vi "Periodic Tasks.vi"(8 "error in":errorcluster) -> ()   [LabVIEW 2013]
doc: "This VI runs in parallel to other tasks. It can contain as many user-defined periodic loops as you need. These can carry out PID or other sorts of timed response."
uses:
  <vilib>/Rock Robotics/SystemInterfaces/DIO/FPGA_DIOChannel.ctl
  <vilib>/Rock Robotics/SystemInterfaces/DIO/FPGA_DIORelayChannel.ctl
  <vilib>/Rock Robotics/SystemInterfaces/Utilities/FPGA_UtilitiesLED Source.ctl
  <vilib>/Rock Robotics/SystemInterfaces/Utilities/FPGA_UtilitiesLED State.ctl
  871/Utils/Targetsss.ctl
  871/Utils/Target Type.ctl
  871/Utils/Scores.ctl
  <vilib>/Rock Robotics/WPI/Counter/WPI_CounterDigitalInputToDigitalSource.vi
  Robot Global Data.vi
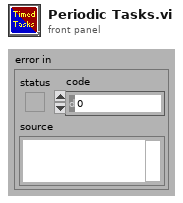
[diagram p1: front panel]
types:
  T1 = typedef "FPGA_DIORelayChannel.ctl" = enum8{"Relay 1", "Relay 2", "Relay 3", "Relay 4", "Relay 5", "Relay 6", "Relay 7", "Relay 8", "Invalid"}
  T2 = typedef "FPGA_DIOChannel.ctl" = enum8{"DIO 1", "DIO 2", "DIO 3", "DIO 4", "DIO 5", "DIO 6", "DIO 7", "DIO 8", "DIO 9", "DIO 10", "DIO 11", "DIO 12", "DIO 13", "DIO 14", "Invalid"}
  T3 = typedef "WPI_DigitalInputDevRef.ctl" = cluster{"DevStatus":errorcluster, "DIO Channel":T2, "Digital Module":T4}
  T4 = typedef "FPGA_TypedefDigitalModule.ctl" = enum16{"Digital Module 1", "Digital Module 2"}
  T5 = typedef "FPGA_CounterEncoderSourceConvertionLVSourceType.ctl" = cluster{"DevStatus":errorcluster, "AnalogTriggerMode?":bool, "DigitalMode":cluster{"Digital Module":T4, "DIO Channel":T6}, "AnalogTriggerMode":cluster{"AnalogTriggerIndex":T7, "OutputType":T8}}
  T6 = typedef "FPGA_DIODigitalSourceChannel.ctl" = enum8{"DIO 1", "DIO 2", "DIO 3", "DIO 4", "DIO 5", "DIO 6", "DIO 7", "DIO 8", "DIO 9", "DIO 10", "DIO 11", "DIO 12", "DIO 13", "DIO 14", "Disabled"}
  T7 = typedef "FPGA_AnalogTriggerIndex.ctl" = enum8{"Trig 0", "Trig 1", "Trig 2", "Trig 3", "Trig 4", "Trig 5", "Trig 6", "Trig 7", "Invalid"}
  T8 = typedef "FPGA_AnalogTriggerOutType.ctl" = enum16{"InWindow", "TriggerState", "Rising", "Falling"}
  T9 = typedef "WPI_InterruptRef.ctl" = cluster{"DevStatus":errorcluster, "InterruptIndex":T10}
  T10 = typedef "FPGA_InterruptIndex.ctl" = enum8{"0", "1", "2", "3", "4", "5", "6", "7", "Invalid"}
  T11 = typedef "FPGA_UtilitiesLED State.ctl" = enum16{"Off", "On", "Toggle"}
  T12 = typedef "FPGA_UtilitiesLED Source.ctl" = enum16{"User LED", "FPGA LED"}
  T13 = typedef "Targetsss.ctl" = cluster{"Vertical Target":T14, "Horizontal Target":T14, "Valid?":bool, "Scores":T15, "Hot?":bool}
  T14 = typedef "Target Type.ctl" = cluster{"Area":dbl, "Bounding box":cluster{"BB Left":dbl, "BB Top":dbl, "BB Right":dbl, "BB Bottom":dbl}, "Center of Mass":cluster{"X Value":dbl, "Y Value":dbl}, "Equivilent Rectangle":cluster{"Width":dbl, "Height":dbl}, "Aspect Ratio":dbl, "Rectangularity":dbl, "Horizontal?":bool}
  T15 = typedef "Scores.ctl" = cluster{"Score Total":dbl, "Left Score":dbl, "Right Score":dbl, "Vertical Score":dbl, "Index":dbl}
  T16 = typedef "WPI_CompressorDevRef.ctl" = cluster{"DevStatus":errorcluster, "DigitalInputDevRef":T3, "RelayDevRef":T17}
  T17 = typedef "WPI_RelayDevRef.ctl" = cluster{"DevStatus":errorcluster, "Relay Channel":T1, "Digital Module":T4, "Relay Direction":T18}
  T18 = typedef "WPI_RelayDirection.ctl" = enum16{"Both directions", "Forward only", "Reverse only"}
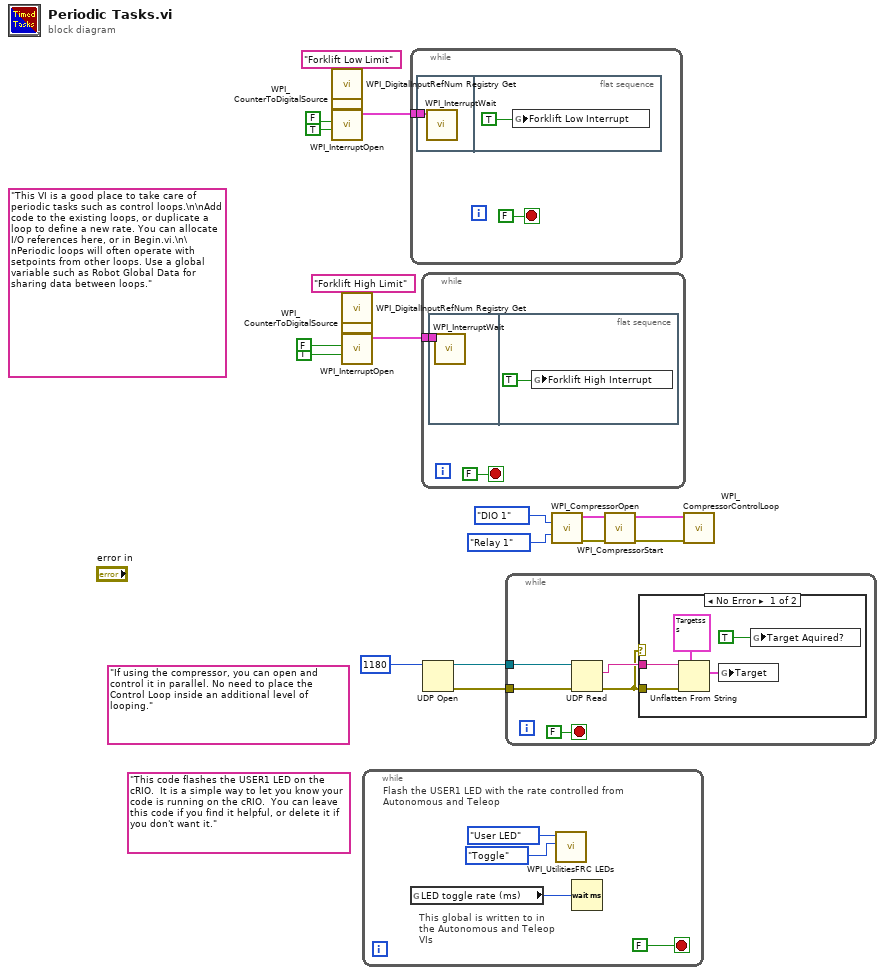
[diagram p0: block diagram]
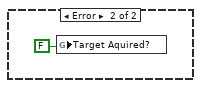
[diagram p2: hidden frame]
diagram:
  (unwired) "If using the compressor, you can open and control it in parallel. No need to place the Control Loop inside an additional level of looping."
  (unwired) "This code flashes the USER1 LED on the cRIO.  It is a simple way to let you know your code is running on the cRIO.  You can leave this code if you find it helpful, or delete it if you don't want it."
  (unwired) "This VI is a good place to take care of periodic tasks such as control loops.\n\nAdd code to the existing loops, or duplicate a loop to define a new rate. You can allocate I/O references here, or in Begin.vi.\n\nPeriodic loops will often operate with setpoints from other loops. Use a global variable such as Robot Global Data for sharing data between loops."
  n1 = call <vilib>:"WPI_DigitalInputRefNum Registry Get.vi"("refnum name"="Forklift Low Limit") -> ("DigitalInputDevRef"=w7:T3)  [unwired: 9 in, 1 out]
  n2 = call-poly <vilib>:"WPI_CounterToDigitalSource.vi"("DigitalInputDevRef"=w7) -> ("Digital Source"=w6:T5)  [unwired: 6 in]
  n3 = call <vilib>:"WPI_InterruptOpen.vi"("Falling Edge"=TRUE, "Rising Edge"=FALSE, "Source"=w6) -> ("InterruptRef"=w5:T9)  [unwired: 7 in, 1 out]
  n4 = call <vilib>:"WPI_DigitalInputRefNum Registry Get.vi"("refnum name"="Forklift High Limit") -> ("DigitalInputDevRef"=w11:T3)  [unwired: 9 in, 1 out]
  n5 = call-poly <vilib>:"WPI_CounterToDigitalSource.vi"("DigitalInputDevRef"=w11) -> ("Digital Source"=w10:T5)  [unwired: 6 in]
  n6 = call <vilib>:"WPI_InterruptOpen.vi"("Falling Edge"=TRUE, "Rising Edge"=FALSE, "Source"=w10) -> ("InterruptRef"=w9:T9)  [unwired: 7 in, 1 out]
  n7 = while {
    stop <- FALSE stop-if-true
    # "This global is written to in the Autonomous and Teleop VIs"
    # "Flash the USER1 LED with the rate controlled from Autonomous and Teleop"
    n8 = global read "Robot Global Data.vi" "LED toggle rate (ms)"() -> (w22:u32)
    n9 = call <vilib>:"WPI_UtilitiesFRC LEDs.vi"("State"=FPGA_UtilitiesLED_State."Toggle", "LED Type"=FPGA_UtilitiesLED_Source."User LED") -> ()  [unwired: 1 in, 9 out]
    n10 = Wait (ms)(milliseconds to wait=w22) -> ()  [unwired: 1 out]
  }
  n11 = while {
    tunnel: w5 -> [w26]
    stop <- FALSE stop-if-true
    n12 = flat-sequence {
      tunnel: w26 -> [w28]
      frame #0 {
        n13 = call <vilib>:"WPI_InterruptWait.vi"("InterruptRef"=w28) -> ()  [unwired: 7 in, 4 out]
      }
      frame #1 {
        n14 = global write "Robot Global Data.vi" "Forklift Low Interrupt"(TRUE) -> ()
      }
    }
  }
  n15 = while {
    tunnel: w9 -> [w30]
    stop <- FALSE stop-if-true
    n16 = flat-sequence {
      tunnel: w30 -> [w32]
      frame #0 {
        n17 = call <vilib>:"WPI_InterruptWait.vi"("InterruptRef"=w32) -> ()  [unwired: 7 in, 4 out]
      }
      frame #1 {
        n18 = global write "Robot Global Data.vi" "Forklift High Interrupt"(TRUE) -> ()
      }
    }
  }
  n19 = UDP Open(11:1180) -> (port=w20:refnum<k16>, 0:w19:errorcluster)  [unwired: 4 in, 1 out]
  n20 = while {
    tunnel: w20 -> [w37]
    tunnel: w19 -> [w36]
    stop <- FALSE stop-if-true
    n21 = UDP Read(connection ID=w37, 8:w36) -> (data out=w35:string, error out=w34:errorcluster)  [unwired: 2 in, 3 out]
    n22 = case shown="No Error" w34 {
      tunnel: w35 -> [w43 _]
      tunnel: w34 -> [w42 _]
      frame No Error {
        n23 = Unflatten From String(type=T13 {"Vertical Target"={"Area"=0.0, "Bounding box"={"BB Left"=0.0, "BB Top"=0.0, "BB Right"=0.0, "BB Bottom"=0.0}, "Center of Mass"={"X Value"=0.0, "Y Value"=0.0}, "Equivilent Rectangle"={"Width"=0.0, "Height"=0.0}, "Aspect Ratio"=0.0, "Rectangularity"=0.0, "Horizontal?"=FALSE}, "Horizontal Target"={"Area"=0.0, "Bounding box"={"BB Left"=0.0, "BB Top"=0.0, "BB Right"=0.0, "BB Bottom"=0.0}, "Center of Mass"={"X Value"=0.0, "Y Value"=0.0}, "Equivilent Rectangle"={"Width"=0.0, "Height"=0.0}, "Aspect Ratio"=0.0, "Rectangularity"=0.0, "Horizontal?"=FALSE}, "Valid?"=FALSE, "Scores"={"Score Total"=0.0, "Left Score"=0.0, "Right Score"=0.0, "Vertical Score"=0.0, "Index"=0.0}, "Hot?"=FALSE} ("Targetssssss"), binary string=w43, error in (no error)=w42) -> (value=w41:T13)  [unwired: 2 in, 2 out]
        n24 = global write "Robot Global Data.vi" "Target"(w41) -> ()
        n25 = global write "Robot Global Data.vi" "Target Aquired?"(TRUE) -> ()
      }
      frame Error {
        n26 = global write "Robot Global Data.vi" "Target Aquired?"(FALSE) -> ()
      }
    }
  }
  n27 = call <vilib>:"WPI_CompressorOpen.vi"("Pressure Switch DIO Channel"=FPGA_DIOChannel."DIO 1" ("DIO Channel"), "Relay Channel"=FPGA_DIORelayChannel."Relay 1") -> ("CompressorDevRef"=w18:T16, "error out"=w15:errorcluster)  [unwired: 12 in]
  n28 = call <vilib>:"WPI_CompressorStart.vi"("error in (no error)"=w15, "CompressorDevRef"=w18) -> ("error out"=w16:errorcluster, "CompressorDevRef"=w17:T16)  [unwired: 8 in]
  n29 = call <vilib>:"WPI_CompressorControlLoop.vi"("error in (no error)"=w16, "CompressorDevRef"=w17) -> ()  [unwired: 10 in]
